vi "Write stream.enabled.vi"(8 "error in (no error)":errorcluster, 10 "stream.enabled":bool, 11 "7976R_v1 in":refnum<class "7976R_v1.lvclass">) -> (0 "error out":errorcluster, 3 "7976R_v1 out":refnum<class "7976R_v1.lvclass">)   [LabVIEW 2015, in "7976R_v1.lvclass"]
uses:
  <userlib>/SE-APP-Receiver/NI5772/7976R_v1/7976R_v1.lvclass
  <userlib>/SE-APP-Receiver/NI5772/7976R_v1/7976R_v1.lvclass/7976R_v1.ctl
  <vilib>/Utility/error.llb/Error Cluster From Error Code.vi
  <vilib>/rvi/errors/niLvFpgaAdjustHostInterfaceError.vi
  <vilib>/rvi/interface/nirviReadWriteControl/nirviReadWriteControl.xnode
  <userlib>/SE-APP-Receiver/NI5772/7976R_v1/Private/FPGA VI Reference_DDC_v1.8.ctl
  NiFpgaLv.dll
  <vilib>/rvi/interface/Simulation/niFpgaSimulationCallBeginRW.vi
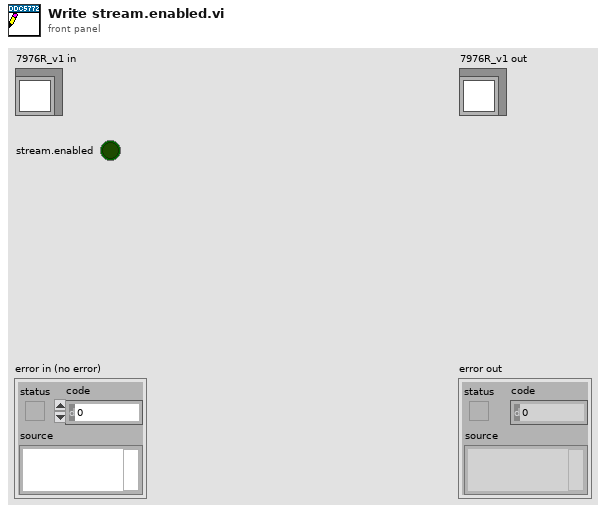
[diagram p1: front panel]
types:
  T1 = typedef "7976R_v1.lvclass/FPGA VI Reference_DDC_v1.8.ctl" = refnum<k20>
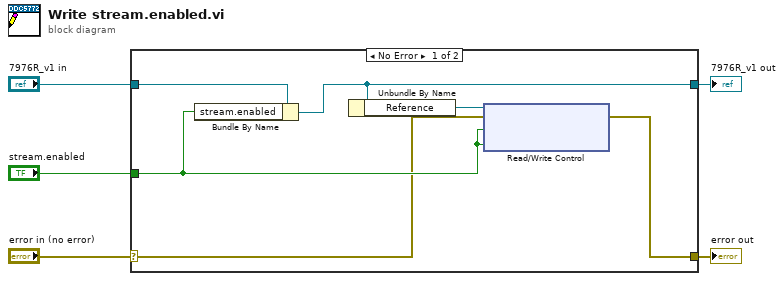
[diagram p0: block diagram]
diagram:
  n1 = case shown="No Error" "error in (no error)" {
    selector: "error in (no error)" -> [w7 w12]
    tunnel: [w6 w12] -> w4
    tunnel: [w10 w13] -> w2
    tunnel: "7976R_v1 in" -> [w11 w13]
    tunnel: "stream.enabled" -> [w8 _]
    frame No Error {
      n2 = Bundle By Name(cluster=w11, "stream.enabled"=w8) -> (w10:refnum<class "7976R_v1.lvclass">)
      n3 = Unbundle By Name(w10) -> ("Reference"=w9:T1)
      n4 = xnode "Read/Write Control"("FPGA VI Reference In"=w9, "error in"=w7, "dbg.stream.enable.2"=w8, "dbg.stream.enable.1"=w8) -> ("error out"=w6:errorcluster)  [unwired: 1 out]
    }
    frame Error {
    }
  }
  "error out" <- w4
  "7976R_v1 out" <- w2
